vi "Return X Position of Cursors iso.vi"(11 "WaveformGraph in":refnum<vi>) -> (1 "After pull Cursor Position":dbl, 2 "Before Pull Cursor Position":dbl, 3 "SW Cursor Position":dbl)   [LabVIEW 2016]
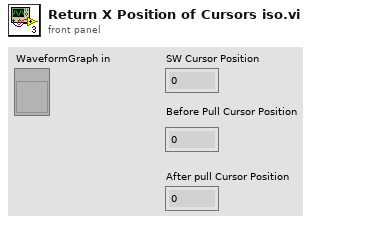
[diagram p1: front panel]
types:
  T1 = typedef "LVCursorListTypeDef.ctl" = cluster{"Name":string, "Color":u32, "Style":u8, "Point Style":u8, "Name Visible":bool, "Allow Drag":bool, "Cursor Mode":u32, "Plot":i32, "Index":i32, "Position":cluster{"X":dbl, "Y":dbl}, "X Scale":u32, "Y Scale":u32, "Watch Plots":i32[], "Watch All Plots":bool, "Plot Area":i32, "Label Offset":cluster{"X":dbl, "Y":dbl}}[]
  T2 = cluster{"Name":string, "Color":u32, "Style":u8, "Point Style":u8, "Name Visible":bool, "Allow Drag":bool, "Cursor Mode":u32, "Plot":i32, "Index":i32, "Position":cluster{"X":dbl, "Y":dbl}, "X Scale":u32, "Y Scale":u32, "Watch Plots":i32[], "Watch All Plots":bool, "Plot Area":i32, "Label Offset":cluster{"X":dbl, "Y":dbl}}
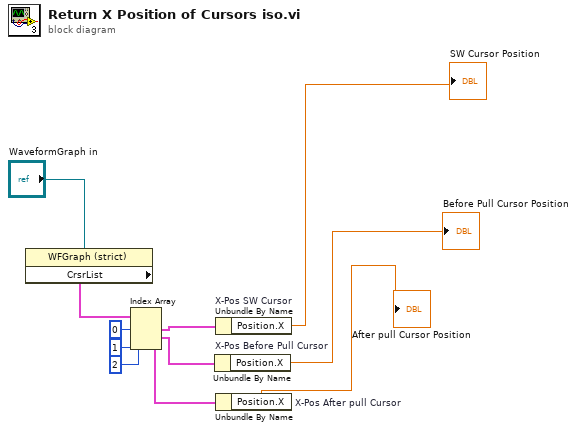
[diagram p0: block diagram]
diagram:
  n1 = property on="Property Node" class="WFGraph (strict)"(reference="WaveformGraph in") -> ("CrsrList"=w1:T1)  [unwired: 1 in, 2 out]
  n2 = Index Array(array=w1, index #1=0 ("index"), index #2=1 ("index"), index #3=2 ("index")) -> (element #1=w6:T2, element #2=w7:T2, element #3=w8:T2)
  n3 = Unbundle By Name "X-Pos Before Pull Cursor"(w7) -> ("Position.X"=→"Before Pull Cursor Position":dbl)
  n4 = Unbundle By Name "X-Pos SW Cursor"(w6) -> ("Position.X"=→"SW Cursor Position":dbl)
  n5 = Unbundle By Name "X-Pos After pull Cursor"(w8) -> ("Position.X"=→"After pull Cursor Position":dbl)
